vi "KE6221 -- Get PDelta Power Meas Type.vi"(0 "6221 Resource In":refnum<visa-resource-name>, 1 "Check For SCPI Errors? (T)":bool=TRUE, 11 "error in (no error)":errorcluster) -> (4 "6221 Resource Out (dupl)":refnum<visa-resource-name>, 8 "Power Meas Type":T1, 15 "error out":errorcluster)   [LabVIEW 2019, in "Keithley 622x.lvlib"]
doc: "Returns the power measurement type that will be returned for 'Pulsed Delta' measurements (Average or Peak). This VI can only be used with a 6221 since the 6220 doesn't support 'Pulsed Delta' measurements. In addition, it is assumed that a 2182/2182A is connected to the 6221 to perform the acutal measurementss (i.e. the 6221 has no measurement capability)."
uses:
  Keithley 622x.lvlib
  Typedefs/KE6221 -- PDelta Power Meas Type.ctl
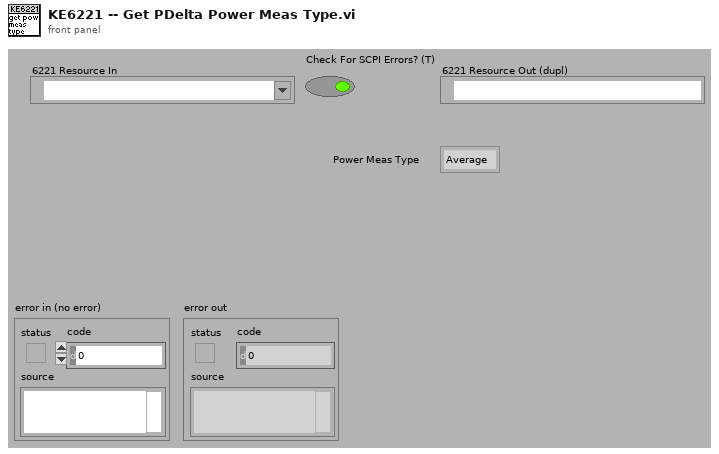
[diagram p1: front panel]
types:
  T1 = typedef "Keithley 622x.lvlib/KE6221 -- PDelta Power Meas Type.ctl" = enum16{"Average", "Peak"}
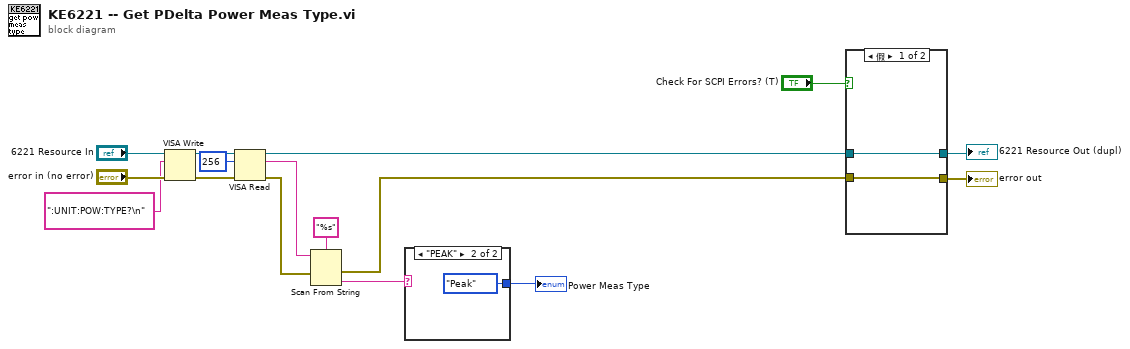
[diagram p0: block diagram]
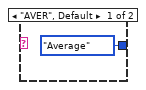
[diagram p2: hidden frame]
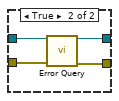
[diagram p3: hidden frame]
diagram:
  n1 = VISA Write(VISA resource name="6221 Resource In", write buffer=":UNIT:POW:TYPE?\n" ("format string"), error in (no error)="error in (no error)") -> (VISA resource name out=w10:refnum<visa-resource-name>, error out=w9:errorcluster)  [unwired: 1 out]
  n2 = VISA Read(VISA resource name=w10, byte count=u32 256, error in (no error)=w9) -> (VISA resource name out=w7:refnum<visa-resource-name>, read buffer=w3:string, error out=w6:errorcluster)  [unwired: 1 out]
  n3 = Scan From String(format string="%s", input string=w3, error in=w6) -> (error out=w5:errorcluster, output 1=w2:string)  [unwired: 2 in, 2 out]
  n4 = case shown="\"PEAK\"" w2 {
    tunnel: [KE6221_--_PDelta_Power_Meas_Type."Average" ("Power Meas Type") KE6221_--_PDelta_Power_Meas_Type."Peak" ("Power Meas Type")] -> w1
    frame "AVER", Default {
    }
    frame "PEAK" {
    }
  }
  "Power Meas Type" <- w1
  n5 = case shown="假" "Check For SCPI Errors? (T)" {
    tunnel: w7 -> [w20 w24]
    tunnel: w5 -> [w19 w23]
    tunnel: [w19 w22] -> w12
    tunnel: [w20 w21] -> w13
    frame False {
    }
    frame True {
      n6 = call "Error Query.vi"("VISA Resource In"=w24, "error in (no error)"=w23) -> ("VISA Resource Out (dupl)"=w21:refnum<visa-resource-name>, "error out"=w22:errorcluster)  [unwired: 10 in, 2 out]
    }
  }
  "6221 Resource Out (dupl)" <- w13
  "error out" <- w12
